vi "MedianFilter.vi"(8 "last array 2":dbl[][](array[numeric]), 11 "Waveform Chart":dbl[][](array[numeric])) -> (1 "output array":dbl[][](array[numeric]))   [LabVIEW 2016]
uses:
  <vilib>/Analysis/NI_AALBase.lvlib
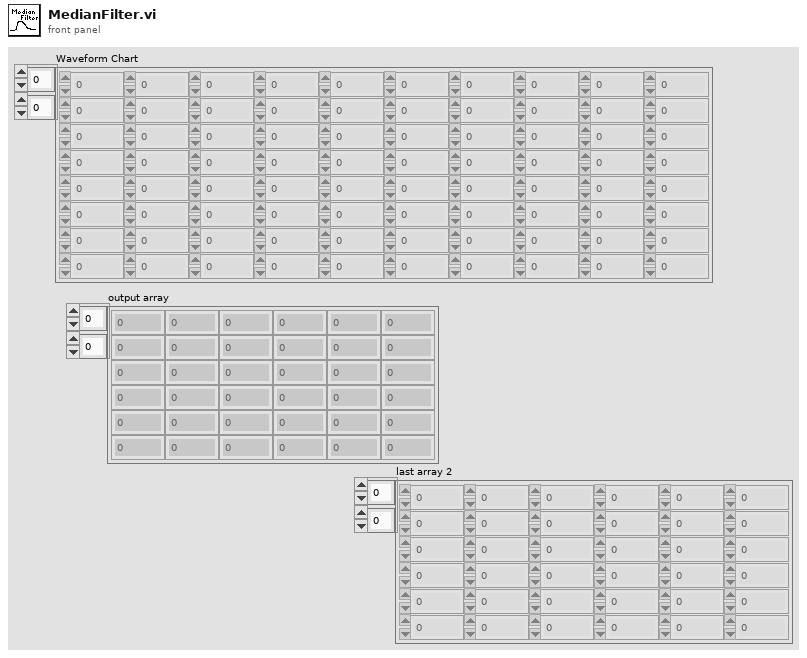
[diagram p1: front panel]
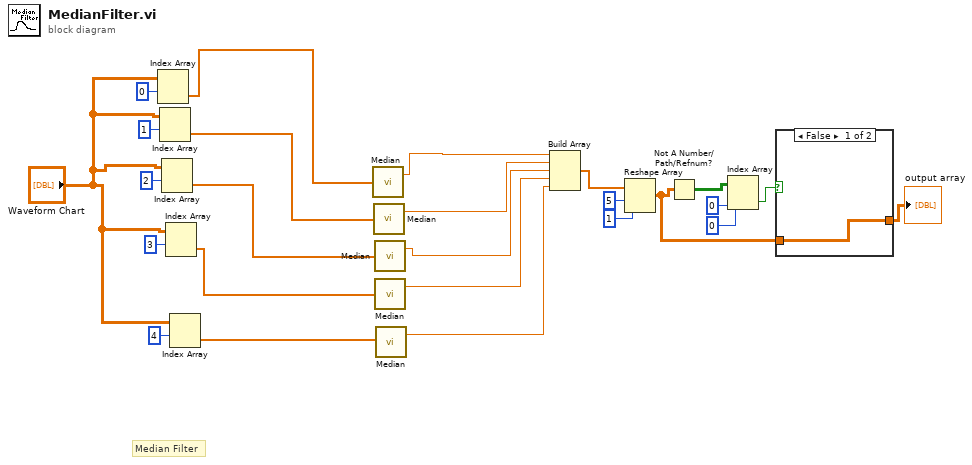
[diagram p0: block diagram]
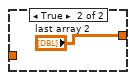
[diagram p2: hidden frame]
diagram:
  # "Median Filter"
  n1 = Index Array(array="Waveform Chart", index (row)=0) -> (element=w21:dbl[])  [unwired: 1 in]
  n2 = Index Array(array="Waveform Chart", index (row)=1) -> (element=w20:dbl[])  [unwired: 1 in]
  n3 = Index Array(array="Waveform Chart", index (row)=2) -> (element=w19:dbl[])  [unwired: 1 in]
  n4 = Index Array(array="Waveform Chart", index (row)=3) -> (element=w18:dbl[])  [unwired: 1 in]
  n5 = Index Array(array="Waveform Chart", index (row)=4) -> (element=w2:dbl[])  [unwired: 1 in]
  n6 = call <vilib>:"Median.vi"("X"=w21) -> ("median"=w17:dbl)  [unwired: 1 out]
  n7 = call <vilib>:"Median.vi"("X"=w20) -> ("median"=w16:dbl)  [unwired: 1 out]
  n8 = call <vilib>:"Median.vi"("X"=w19) -> ("median"=w15:dbl)  [unwired: 1 out]
  n9 = call <vilib>:"Median.vi"("X"=w18) -> ("median"=w14:dbl)  [unwired: 1 out]
  n10 = call <vilib>:"Median.vi"("X"=w2) -> ("median"=w1:dbl)  [unwired: 1 out]
  n11 = Build Array(w17, w16, w15, w14, w1) -> (w13:dbl[])
  n12 = Reshape Array(w13, 5 ("dimension size"), 1 ("dimension size")) -> (w5:dbl[][])
  n13 = Not A Number/Path/Refnum?(number/path/refnum=w5) -> (NaN/Path/Refnum?=w10:bool[][])
  n14 = Index Array(array=w10, index (row)=0 ("disabled index (row)"), index (col)=0 ("disabled index (col)")) -> (element=w7:bool)
  n15 = case shown="False" w7 {
    tunnel: [w26 "last array 2"] -> w6
    tunnel: w5 -> [w26 _]
    frame False {
    }
    frame True {
    }
  }
  "output array" <- w6
